vi "Read Rigid Body Data.vi"(8 "error in (no error)":errorcluster, 11 "Tracking Data In":T1) -> (0 "error out":errorcluster, 3 "Tracking Data Out":T1)   [LabVIEW 2017]
uses:
  Controls/Tracking Data Multi Body.ctl
  Controls/Packet Data.ctl
  Controls/Rigid Body Info.ctl
  Controls/Position.ctl
  Controls/Orientation.ctl
  Controls/Tracker Type.ctl
panel:
  out "Rigid Bodies":T3[](array[typedef])
  out "return count":u32
  out "read buffer":string
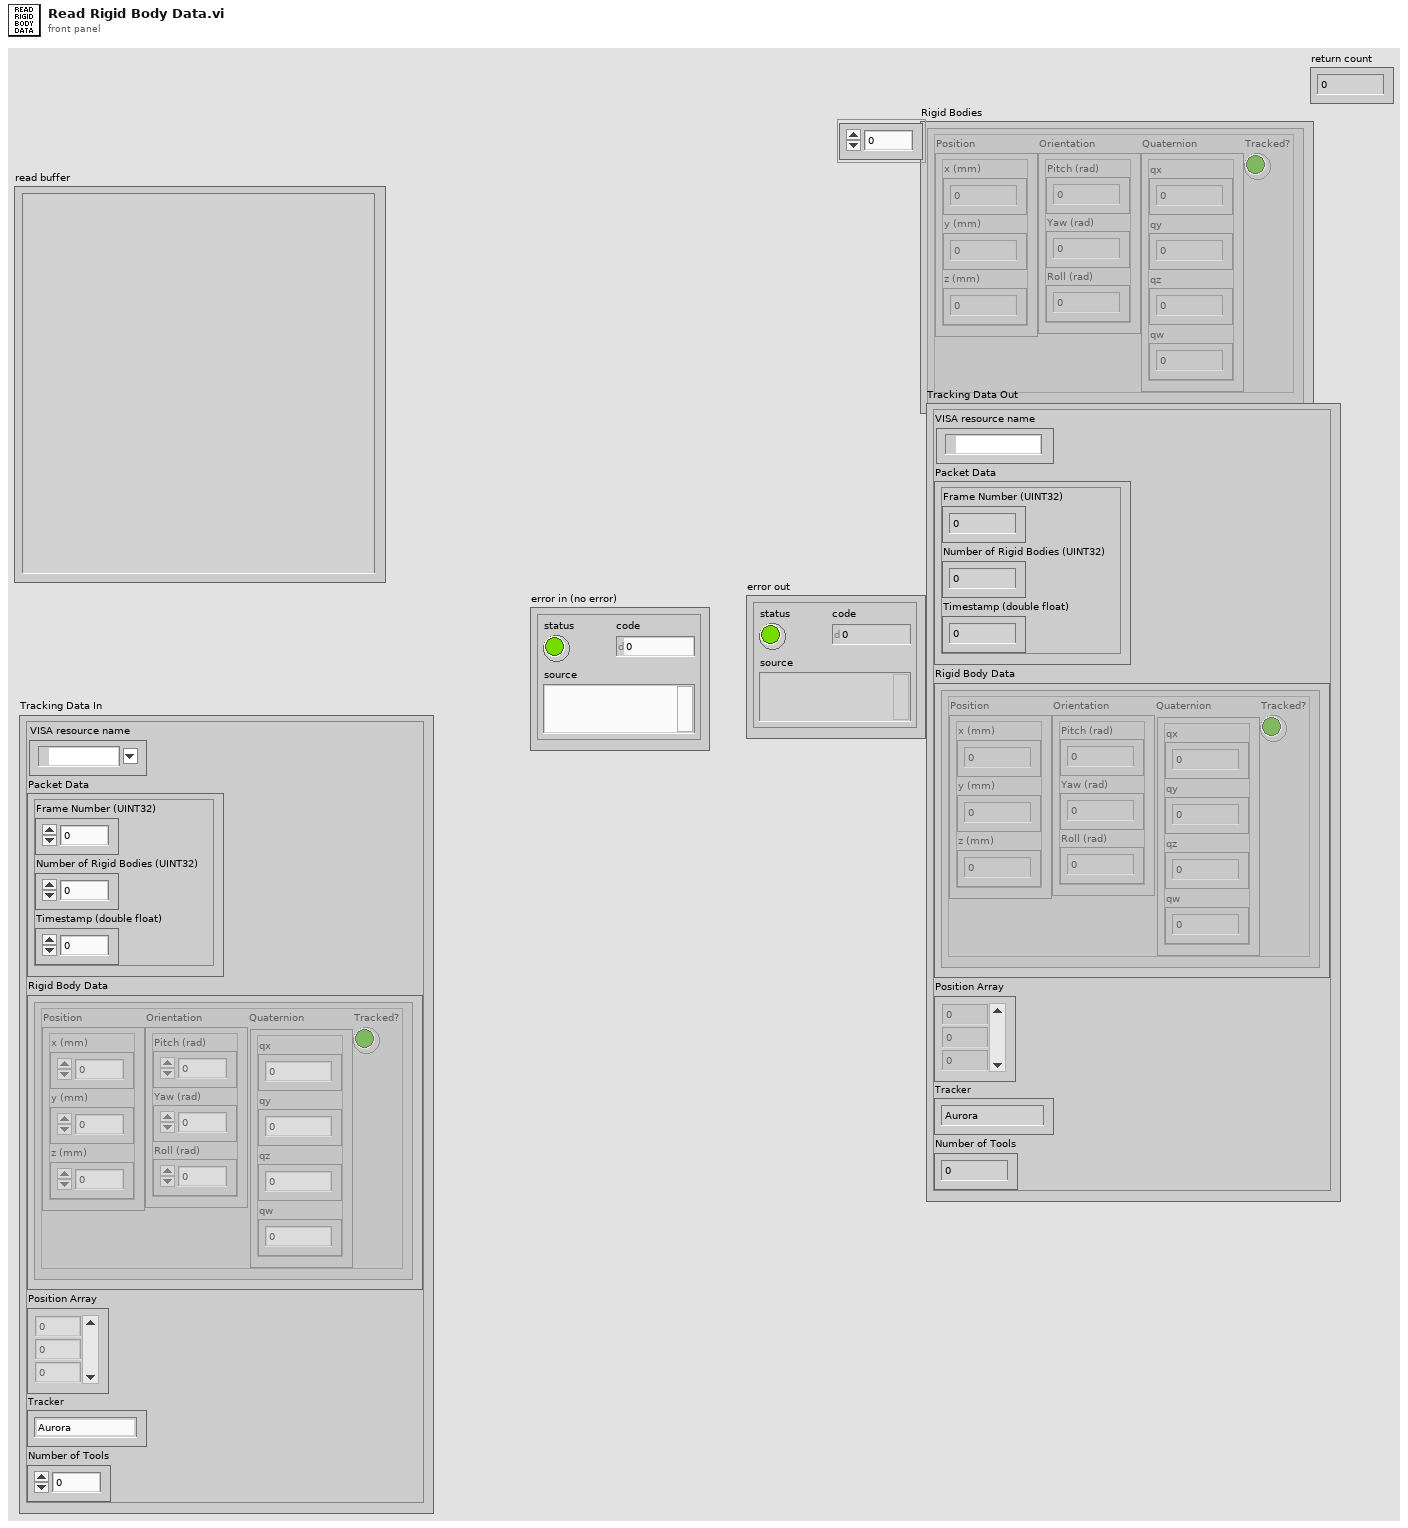
[diagram p1: front panel]
types:
  T1 = typedef "Tracking Data Multi Body.ctl" = cluster{"VISA resource name":refnum<visa-resource-name>, "Packet Data":T2, "Rigid Body Data":T3[], "Position Array":dbl[][], "Tracker":T6, "Number of Tools":u32}
  T2 = typedef "Packet Data.ctl" = cluster{"Frame Number (UINT32)":u32, "Number of Rigid Bodies (UINT32)":u32, "Timestamp (double float)":dbl}
  T3 = typedef "Rigid Body Info.ctl" = cluster{"Position":T4, "Orientation":T5, "Quaternion":cluster{"qx":sgl, "qy":sgl, "qz":sgl, "qw":sgl}, "Tracked?":bool}
  T4 = typedef "Position.ctl" = cluster{"x (mm)":sgl, "y (mm)":sgl, "z (mm)":sgl}
  T5 = typedef "Orientation.ctl" = cluster{"Pitch (rad)":sgl, "Yaw (rad)":sgl, "Roll (rad)":sgl}
  T6 = typedef "Tracker Type.ctl" = enum16{"Aurora", "OptiTrack"}
  T7 = typedef "Raw Rigid Body Data.ctl" = cluster{"Body ID (UINT32)":u32, "x (single float)":sgl, "y (single float)":sgl, "z (single float)":sgl, "qx (single float)":sgl, "qy (single float)":sgl, "qz (single float)":sgl, "qw (single float)":sgl, "Tracked 1 (UINT8)":u8, "Tracked 2 (UINT8)":u8}
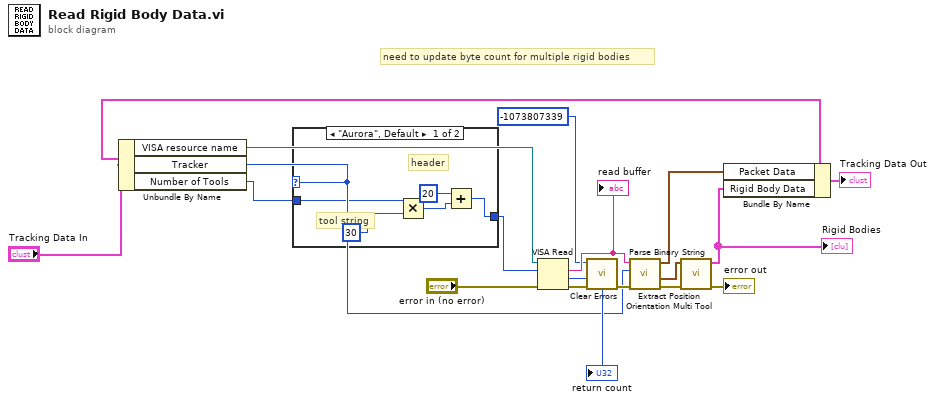
[diagram p0: block diagram]
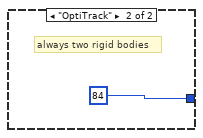
[diagram p2: hidden frame]
diagram:
  # "need to update byte count for multiple rigid bodies"
  n1 = Unbundle By Name("Tracking Data In") -> ("VISA resource name"=w9:refnum<visa-resource-name>, "Tracker"=w3:T6, "Number of Tools"=w1:u32)
  n2 = case shown="\"Aurora\", Default" w3 {
    tunnel: [w18 u32 84 ("byte count")] -> w2
    tunnel: w1 -> [w21 _]
    frame "Aurora", Default {
      # "tool string"
      # "header"
      n3 = Multiply(x=w21, y=u32 30 ("byte count 2")) -> (x*y=w22:u32)
      n4 = Add(x=u32 20, y=w22) -> (x+y=w18:u32)
    }
    frame "OptiTrack" {
      # "always two rigid bodies"
    }
  }
  n5 = VISA Read(VISA resource name=w9, byte count=w2, error in (no error)="error in (no error)") -> (read buffer=w13:string, return count=→"return count":u32, error out=w12:errorcluster)  [unwired: 1 out]
  "read buffer" <- w13
  n6 = call <vilib>:"Clear Errors.vi"("error in (no error)"=w12, "specific error code to clear (0: all)"=-1073807339) -> ("error out"=w14:errorcluster)  [unwired: 4 in, 1 out]
  n7 = call "Parse Binary String.vi"("Error In"=w14, "Tracker"=w3, "read buffer in"=w13) -> ("Error Out"=w16:errorcluster, "Rigid Body Data"=w15:T7[], "Packet Data"=w8:T2)  [unwired: 5 in, 1 out]
  n8 = call "Extract Position Orientation Multi Tool.vi"("Error In"=w16, "Rigid Body Data"=w15) -> ("Error Out"=→"error out":errorcluster, "Rigid Bodies"=w5:T3[])  [unwired: 8 in]
  "Rigid Bodies" <- w5
  n9 = Bundle By Name(cluster="Tracking Data In", "Packet Data"=w8, "Rigid Body Data"=w5) -> (→"Tracking Data Out":T1)
